vi "RSNRPZ Channel Reset.vi"(8 "error in (no error)":errorcluster, 10 "Channel (1)":i32=1, 11 "VISA session":refnum<visa-resource-name> caption="VISA resource name") -> (0 "error out":errorcluster, 3 "dup VISA session":refnum<visa-resource-name> caption="VISA resource name")   [LabVIEW 2010]
doc: "From the point of view of the R&S NRP basic unit, the sensors are stand-alone measuring devices. They communicate with the R&S NRP via a command set complying with SCPI.\nThis VI prompts the basic unit to send an *RST to the respective sensor. Measurements in progress are interrupted.\n\nRemote-control command(s):\nSYSTem:SENSor[1..4]:RESet"
uses:
  rsnrpz_32.dll
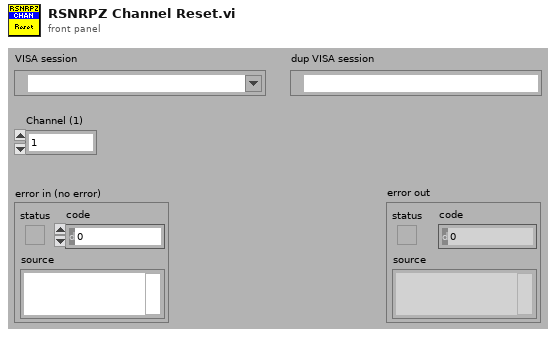
[diagram p1: front panel]
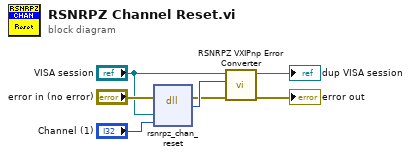
[diagram p0: block diagram]
diagram:
  n1 = dll-call lib="rsnrpz_32.dll" fn="rsnrpz_chan_reset"(error in="error in (no error)", "VISA Session"="VISA session", "Channel"="Channel (1)") -> (error out=w5:errorcluster, "Status"=w7:i32)  [unwired: 4 in, 1 out]
  n2 = call <instrlib>:"RSNRPZ VXIPnp Error Converter.vi"("error in"=w5, "VXIPnp error code"=w7, "VISA session"="VISA session") -> ("error out"=→"error out":errorcluster, "dup VISA session"=→"dup VISA session":refnum<visa-resource-name>)  [unwired: 7 in]
